vi "N 2DGaussianWithRotationFit000.vi"() -> ()   [LabVIEW 2011]
uses:
  <vilib>/gmath/NumericalOptimization/Nonlinear Curve Fit LM.vi
  <vilib>/gmath/NI_Gmath.lvlib
  <vilib>/Analysis/NI_AALBase.lvlib
panel:
  out "Fit":T1(plugin-control)
  out "Data":T1(plugin-control)
  out "number of function calls":i32
  in  "stop":bool
  in  "Simulation":dbl[](array[slide])=[50.0, 10.74766355140187, 12.305295950155763, 2.4922118380062304, 5.14018691588785, 127.10280373831775, 50.0, 19.937694704049843, 5.14018691588785, 3.7383177570093453, 6.853582554517134, 31.61993769470405] caption="Amplitude\n\n\nX-Position\n\n\nY-Position\n\n\nWidth A\n\n\nWidth B\n\n\nAngle\n\n\nAmplitude\n\n\nX-Position\n\n\nY-Position\n\n\nWidth A\n\n\nWidth B\n\n\nAngle" scale=0.0..50.0
  in  "Fit!":bool
  out "Parameters":dbl[][](array[numeric]) caption="Auto Guess                  Actual              Best Fit           Difference" format="%.4f"
  in  "Noise":dbl=10.0
  out "error out":errorcluster
  # "(1) Simulate desired surface by\nchanging parameters and noise\n(2) Press fit and wait a while"
  # "Widths are currently defined as\n2*sigma for code simplicity."
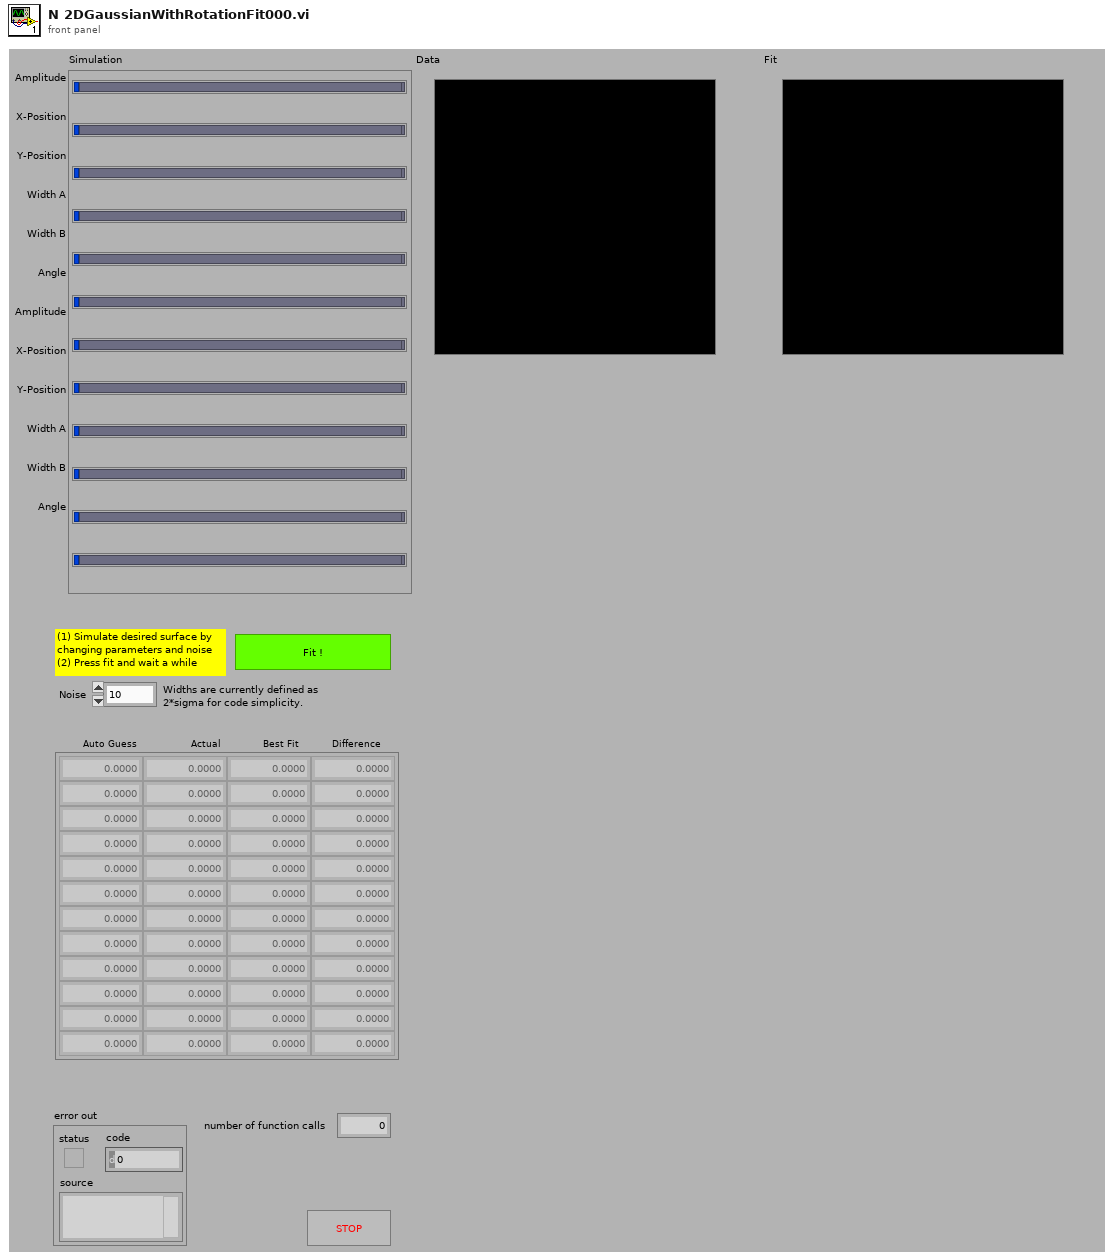
[diagram p1: front panel]
types:
  T1 = typedef "IMAQ Image.ctl" = refnum<image>
  T2 = typedef "Image Type" = u32
  T3 = cluster{"Width":i32, "Height":i32, "N Gaussians":i32}
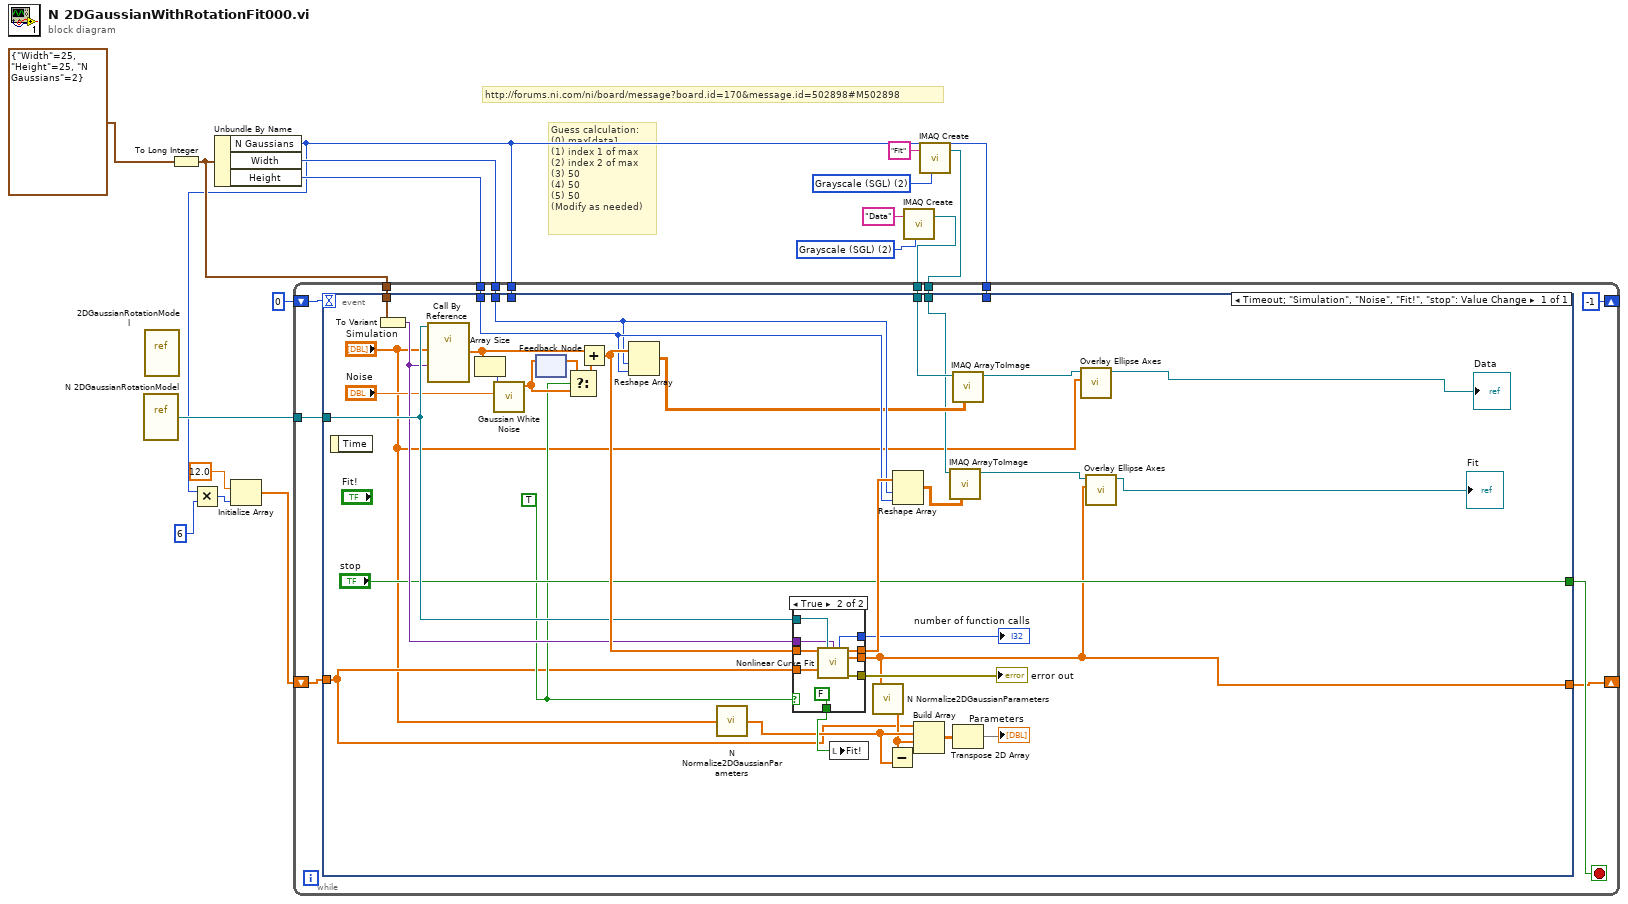
[diagram p0: block diagram]
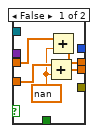
[diagram p2: hidden frame]
diagram:
  w3 = T2 2 items=["Grayscale (U8)", "Grayscale (I16)", "Grayscale (SGL)", "Complex (CSG)", "RGB (U32)", "HSL (U32)", "RGB (U64)", "Grayscale (U16)"] ("Image Type")
  w7 = T2 2 items=["Grayscale (U8)", "Grayscale (I16)", "Grayscale (SGL)", "Complex (CSG)", "RGB (U32)", "HSL (U32)", "RGB (U64)", "Grayscale (U16)"] ("Image Type")
  # "http://forums.ni.com/ni/board/message?board.id=170&message.id=502898#M502898"
  # "Guess calculation:\n(0) max[data]\n(1) index 1 of max\n(2) index 2 of max\n(3) 50\n(4) 50\n(5) 50\n(Modify as needed)"
  n1 = vi-ref "N 2DGaussianRotationModel.vi"() -> (w12:refnum<vi>)
  n2 = vi-ref "2DGaussianRotationModel.vi"() -> ()  [unwired: 1 out]
  n3 = To Long Integer(number=T3 {"Width"=25, "Height"=25, "N Gaussians"=2}) -> (32bit integer=w14:T3)
  n4 = Unbundle By Name(w14) -> ("N Gaussians"=w1:i32, "Width"=w16:i32, "Height"=w15:i32)
  n5 = Multiply(x=w1, y=6 ("dimension size")) -> (x*y=w11:i32)
  n6 = Initialize Array(12.0 ("element"), w11) -> (w8:dbl[])
  n7 = call "IMAQ Create"("Image Name"="Data", "Image Type"=w7) -> ("New Image"=w5:T1)  [unwired: 3 in, 1 out]
  n8 = call "IMAQ Create"("Image Name"="Fit", "Image Type"=w3) -> ("New Image"=w2:T1)  [unwired: 3 in, 1 out]
  n9 = while {
    tunnel: w12 -> [w30]
    tunnel: w14 -> [w29]
    shift-right: [-1] -> _
    shift-left: 0 -> [w26]
    tunnel: w16 -> [w25]
    tunnel: w15 -> [w24]
    tunnel: w1 -> [w23]
    shift-right: [w21] -> _
    shift-left: w8 -> [w22]
    tunnel: w5 -> [w20]
    tunnel: w2 -> [w19]
    tunnel: w1 -> [w18]
    stop <- w28 stop-if-true
    n10 = event shown="[0] Timeout;  \"Simulation\", \"Noise\", \"Fit!\", \"stop\": Value Change" {
      selector: _ -> [_]
      dyn-events: _ -> [_]
      timeout: w26 -> [_]
      tunnel: w30 -> [w57]
      tunnel: w29 -> [w61]
      tunnel: ["stop"] -> w28
      tunnel: w25 -> [w48]
      tunnel: w24 -> [w53]
      tunnel: w23 -> [_]
      tunnel: w22 -> [w41]
      tunnel: [w31] -> w21
      tunnel: w20 -> [w39]
      tunnel: w19 -> [w37]
      tunnel: w18 -> [_]
      event Timeout; "Simulation", "Noise", "Fit!", "stop": Value Change {
        w42 = TRUE
        n11 = event-data() -> ()  [unwired: 1 in, 1 out]
        n12 = To Variant(anything=w61) -> (Variant=w55:variant)
        n13 = call-by-ref "?"(reference=w57, "data"=w55, "a"="Simulation") -> ("f(X,a)"=w56:dbl[])  [unwired: 3 in, 4 out]
        n14 = Array Size(array=w56) -> (size(s)=w63:i32)
        n15 = call <vilib>:"Gaussian White Noise.vi"("standard deviation"="Noise", "samples"=w63) -> ("Gaussian noise pattern"=w51:dbl[])  [unwired: 8 in, 1 out]
        n16 = feedback-in #1(w51) -> ()
        n17 = feedback #1() -> (w50:dbl[])  [unwired: 1 in]
        n18 = Select(t=w50, s=w42, f=w51) -> (s? t:f=w52:dbl[])
        n19 = Add(x=w56, y=w52) -> (x+y=w62:dbl[])
        n20 = Reshape Array(w62, w48, w53) -> (w40:dbl[][])
        n21 = call "N Normalize2DGaussianParameters.vi"("best fit parameters IN"="Simulation") -> ("best fit parameters OUT"=w44:dbl[])
        n22 = case shown="True" w42 {
          tunnel: [w66 w78] -> w64
          tunnel: [_ w77] -> w47
          tunnel: w57 -> [_ w76]
          tunnel: w55 -> [_ w75]
          tunnel: w62 -> [w69 w74]
          tunnel: [w67 w73] -> w31
          tunnel: w41 -> [w68 w72]
          tunnel: [_ w71] -> w49
          tunnel: [_ FALSE] -> w46
          frame False {
            w65 = nan ("element")
            n23 = Add(x=w68, y=w65) -> (x+y=w67:dbl[])
            n24 = Add(x=w69, y=w65) -> (x+y=w66:dbl[])
          }
          frame True {
            n25 = call-poly <vilib>:"Nonlinear Curve Fit.vi"("Y"=w74, "f(x,a)"=w76, "data"=w75, "initial parameters"=w72) -> ("number of function calls"=w71:i32, "best nonlinear fit"=w78:dbl[], "best fit parameters"=w73:dbl[], "error out"=w77:errorcluster)  [unwired: 6 in, 2 out]
          }
        }
        "error out" <- w47
        "number of function calls" <- w49
        n26 = local write "Fit!"(w46) -> ()
        n27 = call "N Normalize2DGaussianParameters.vi"("best fit parameters IN"=w31) -> ("best fit parameters OUT"=w43:dbl[])
        n28 = Subtract(x=w43, y=w44) -> (x-y=w60:dbl[])
        n29 = Reshape Array(w64, w48, w53) -> (w38:dbl[][])
        n30 = Build Array(w41, w44, w43, w60) -> (w59:dbl[][])
        n31 = call "IMAQ ArrayToImage"("Image Pixels (Float)"=w38, "Image"=w37) -> ("Image Out"=w33:T1)  [unwired: 8 in, 1 out]
        n32 = call "IMAQ ArrayToImage"("Image Pixels (Float)"=w40, "Image"=w39) -> ("Image Out"=w36:T1)  [unwired: 8 in, 1 out]
        n33 = Transpose 2D Array(2D array=w59) -> (transposed array=→"Parameters":dbl[][])
        n34 = call "Overlay Ellipse Axes.vi"("array"="Simulation", "Image Out"=w36) -> ("Image Out 2"=→"Data":T1)  [unwired: 9 in]
        n35 = call "Overlay Ellipse Axes.vi"("array"=w31, "Image Out"=w33) -> ("Image Out 2"=→"Fit":T1)  [unwired: 9 in]
      }
    }
  }
